vi "Error Converter (ErrCode or Status).vi"(8 "error in (no error)":errorcluster, 11 "error code":i32) -> (0 "error out":errorcluster)   [LabVIEW 2010]
panel:
  in  "error message (\"\")":string
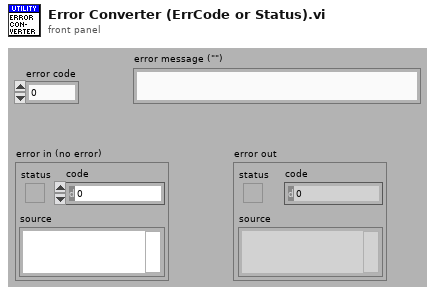
[diagram p1: front panel]
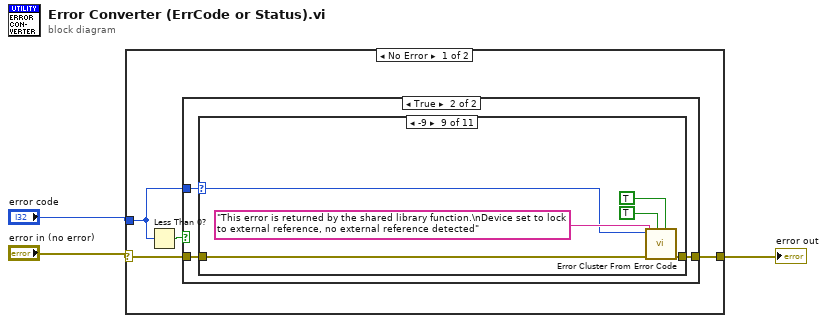
[diagram p0: block diagram]
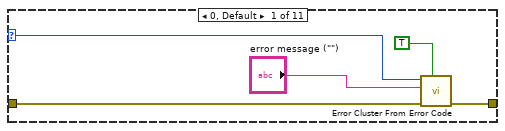
[diagram p3: hidden frame]
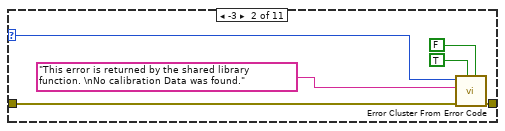
[diagram p4: hidden frame]
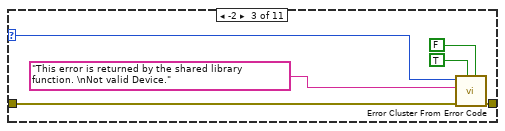
[diagram p5: hidden frame]
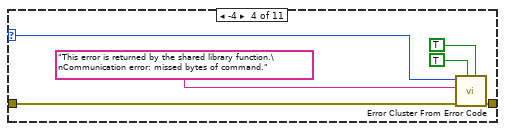
[diagram p6: hidden frame]
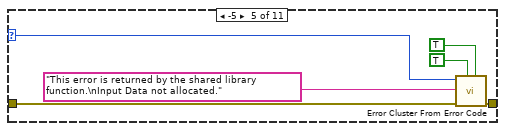
[diagram p7: hidden frame]
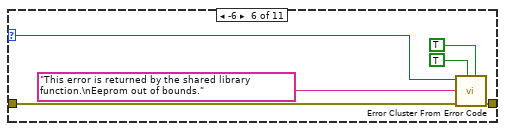
[diagram p8: hidden frame]
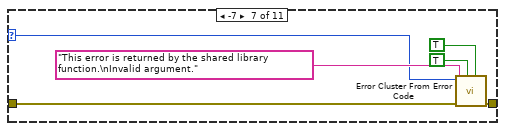
[diagram p9: hidden frame]
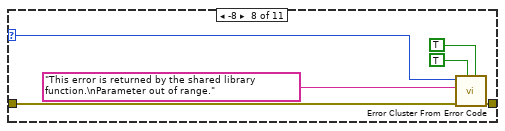
[diagram p10: hidden frame]
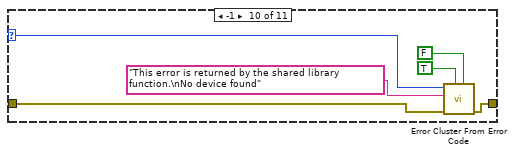
[diagram p11: hidden frame]
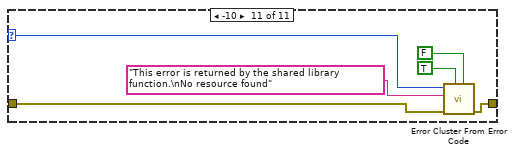
[diagram p12: hidden frame]
diagram:
  n1 = case shown="No Error" "error in (no error)" {
    selector: "error in (no error)" -> [w6 w77]
    tunnel: [w5 w77] -> w1
    tunnel: "error code" -> [w4 _]
    frame No Error {
      n2 = Less Than 0?(x=w4) -> (x < 0?=w7:bool)
      n3 = case shown="True" w7 {
        tunnel: w6 -> [w8 w11]
        tunnel: [w8 w10] -> w5
        tunnel: w4 -> [_ w9]
        frame False {
        }
        frame True {
          n4 = case shown="-9" w9 {
            selector: w9 -> [w12 w19 w25 w30 w36 w42 w48 w54 w60 w68 w74]
            tunnel: w11 -> [w15 w22 w28 w34 w40 w46 w52 w58 w64 w67 w73]
            tunnel: [w14 w21 w27 w33 w39 w45 w51 w57 w63 w65 w71] -> w10
            frame 0, Default {
              n5 = call <vilib>:"Error Cluster From Error Code.vi"("show call chain? (False)"=TRUE, "error in (no error)"=w15, "error message (\"\")"="error message (\"\")", "error code (0)"=w12) -> ("error out"=w14:errorcluster)  [unwired: 5 in]
            }
            frame -3 {
              n6 = call <vilib>:"Error Cluster From Error Code.vi"("is warning? (False)"=FALSE, "show call chain? (False)"=TRUE, "error in (no error)"=w22, "error message (\"\")"="This error is returned by the shared library function. \nNo calibration Data was found." ("string"), "error code (0)"=w19) -> ("error out"=w21:errorcluster)  [unwired: 4 in]
            }
            frame -2 {
              n7 = call <vilib>:"Error Cluster From Error Code.vi"("is warning? (False)"=FALSE, "show call chain? (False)"=TRUE, "error in (no error)"=w28, "error message (\"\")"="This error is returned by the shared library function. \nNot valid Device." ("string"), "error code (0)"=w25) -> ("error out"=w27:errorcluster)  [unwired: 4 in]
            }
            frame -4 {
              n8 = call <vilib>:"Error Cluster From Error Code.vi"("is warning? (False)"=TRUE, "show call chain? (False)"=TRUE, "error in (no error)"=w34, "error message (\"\")"="This error is returned by the shared library function.\nCommunication error: missed bytes of command." ("string 2"), "error code (0)"=w30) -> ("error out"=w33:errorcluster)  [unwired: 4 in]
            }
            frame -5 {
              n9 = call <vilib>:"Error Cluster From Error Code.vi"("is warning? (False)"=TRUE, "show call chain? (False)"=TRUE, "error in (no error)"=w40, "error message (\"\")"="This error is returned by the shared library function.\nInput Data not allocated." ("string 3"), "error code (0)"=w36) -> ("error out"=w39:errorcluster)  [unwired: 4 in]
            }
            frame -6 {
              n10 = call <vilib>:"Error Cluster From Error Code.vi"("is warning? (False)"=TRUE, "show call chain? (False)"=TRUE, "error in (no error)"=w46, "error message (\"\")"="This error is returned by the shared library function.\nEeprom out of bounds." ("string 4"), "error code (0)"=w42) -> ("error out"=w45:errorcluster)  [unwired: 4 in]
            }
            frame -7 {
              n11 = call <vilib>:"Error Cluster From Error Code.vi"("is warning? (False)"=TRUE, "show call chain? (False)"=TRUE, "error in (no error)"=w52, "error message (\"\")"="This error is returned by the shared library function.\nInvalid argument." ("string 5"), "error code (0)"=w48) -> ("error out"=w51:errorcluster)  [unwired: 4 in]
            }
            frame -8 {
              n12 = call <vilib>:"Error Cluster From Error Code.vi"("is warning? (False)"=TRUE, "show call chain? (False)"=TRUE, "error in (no error)"=w58, "error message (\"\")"="This error is returned by the shared library function.\nParameter out of range." ("string 6"), "error code (0)"=w54) -> ("error out"=w57:errorcluster)  [unwired: 4 in]
            }
            frame -9 {
              n13 = call <vilib>:"Error Cluster From Error Code.vi"("is warning? (False)"=TRUE, "show call chain? (False)"=TRUE, "error in (no error)"=w64, "error message (\"\")"="This error is returned by the shared library function.\nDevice set to lock to external reference, no external reference detected" ("string 7"), "error code (0)"=w60) -> ("error out"=w63:errorcluster)  [unwired: 4 in]
            }
            frame -1 {
              n14 = call <vilib>:"Error Cluster From Error Code.vi"("is warning? (False)"=FALSE, "show call chain? (False)"=TRUE, "error in (no error)"=w67, "error message (\"\")"="This error is returned by the shared library function.\nNo device found" ("string 7"), "error code (0)"=w68) -> ("error out"=w65:errorcluster)  [unwired: 4 in]
            }
            frame -10 {
              n15 = call <vilib>:"Error Cluster From Error Code.vi"("is warning? (False)"=FALSE, "show call chain? (False)"=TRUE, "error in (no error)"=w73, "error message (\"\")"="This error is returned by the shared library function.\nNo resource found" ("string 7"), "error code (0)"=w74) -> ("error out"=w71:errorcluster)  [unwired: 4 in]
            }
          }
        }
      }
    }
    frame Error {
    }
  }
  "error out" <- w1
